vi "week5_timer_LV17.vi"() -> ()   [LabVIEW 2017]
panel:
  out "Waveform Chart":dbl(graph)=10.0
  out "Boolean":bool
  out "Progress bar":u8(slide) scale=0.0..10.0
  out "Sequence / Case":bool
  out "Timer count-down [seconds]":dbl format="%.3g"
  in  "Time to wait [seconds]":dbl=5.0
  in  "stop":bool
  # "A"
  # "B"
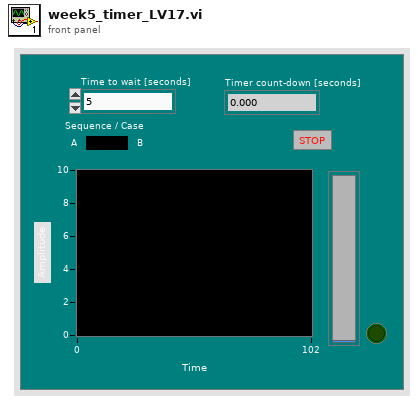
[diagram p1: front panel]
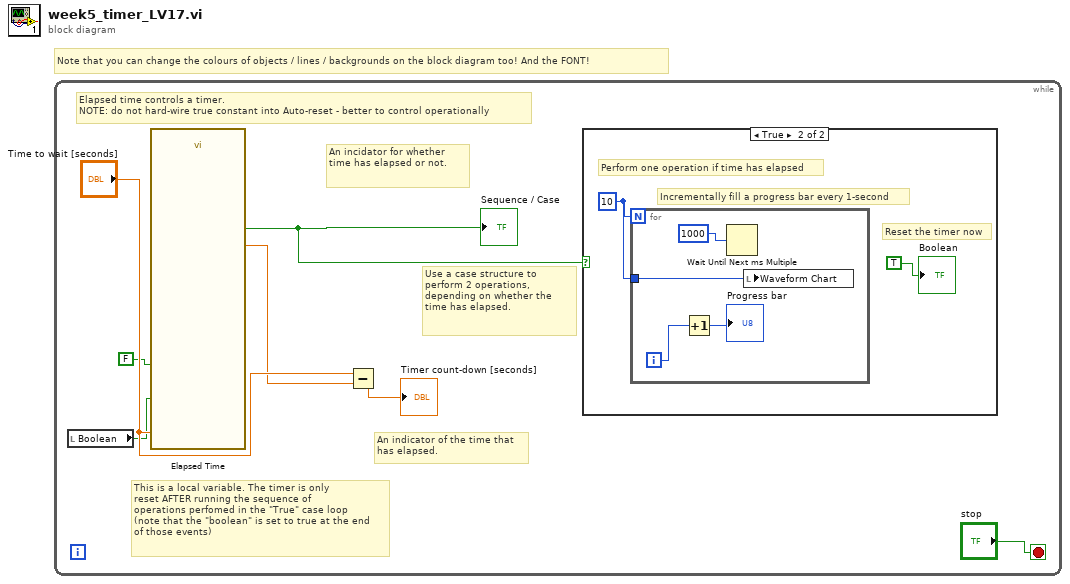
[diagram p0: block diagram]
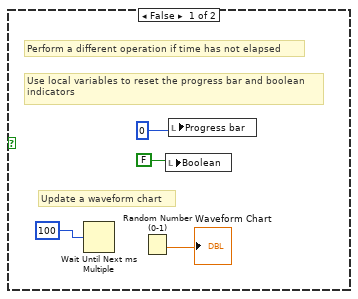
[diagram p2: hidden frame]
diagram:
  # "Note that you can change the colours of objects / lines / backgrounds on the block diagram too! And the FONT!"
  n1 = while {
    stop <- "stop" stop-if-true
    # "This is a local variable. The timer is only \nreset AFTER running the sequence of\noperations perfomed in the \"True\" case loop\n(note that the \"boolean\" is set to true at the end \nof those events)"
    # "Use a case structure to perform 2 operations, \ndepending on whether the time has elapsed."
    # "An incidator for whether time has elapsed or not."
    # "An indicator of the time that\nhas elapsed."
    # "Elapsed time controls a timer. \nNOTE: do not hard-wire true constant into Auto-reset - better to control operationally"
    n2 = local read "Boolean"() -> (w2:bool)
    n3 = call "Elapsed Time"("Time Target (s)"="Time to wait [seconds]", "Reset"=w2, "Auto Reset"=FALSE) -> ("Elapsed Time (s)"=w5:dbl, "Time has Elapsed"=w3:bool)  [unwired: 9 in, 6 out]
    "Sequence / Case" <- w3
    n4 = Subtract(x="Time to wait [seconds]", y=w5) -> (x-y=→"Timer count-down [seconds]":dbl)
    n5 = case shown="True" w3 {
      frame False {
        # "Update a waveform chart"
        # "Use local variables to reset the progress bar and boolean\nindicators"
        # "Perform a different operation if time has not elapsed"
        n6 = Wait Until Next ms Multiple(millisecond multiple=100) -> ()  [unwired: 1 out]
        n7 = Random Number (0-1)() -> (number: 0 to 1=→"Waveform Chart":dbl)
        n8 = local write "Boolean"(FALSE) -> ()
        n9 = local write "Progress bar"(0) -> ()
      }
      frame True {
        w12 = 10
        # "Reset the timer now"
        # "Incrementally fill a progress bar every 1-second"
        # "Perform one operation if time has elapsed"
        n10 = for {
          N: w12 -> [_]
          tunnel: w12 -> [w14]
          i -> [w15]
          n11 = Increment(x=w15) -> (x+1=→"Progress bar":i32)
          n12 = Wait Until Next ms Multiple(millisecond multiple=1000) -> ()  [unwired: 1 out]
          n13 = local write "Waveform Chart"(w14) -> ()
        }
        "Boolean" <- TRUE
      }
    }
  }
